vi "GetPower.vi"(6 "Calculation State in":T5, 8 "error in (no error)":errorcluster, 9 "Channel":T1, 10 "3-phase current waveform":waveform(dbl)[](array[waveform]), 11 "3-phase voltage waveform":waveform(dbl)[](array[waveform])) -> (0 "error out":errorcluster, 2 "power value":T6, 4 "Calculation State out":T5)   [LabVIEW 2017, in "McsaAnalysisFunctions.lvlib"]
uses:
  <vilib>/addons/InsightCM/Utilities/Analysis/MCSA/McsaAnalysisFunctions.lvlib
  <vilib>/addons/InsightCM/Utilities/Analysis/MCSA/controls/MotorCalculationCache.ctl
  <vilib>/addons/Electrical Power/Basic/Measurement/subVIs/basic_Power Value.ctl
  <vilib>/addons/InsightCM/Utilities/Analysis/MCSA/controls/TorqueLoadEfficiency.ctl
  <vilib>/addons/InsightCM/Utilities/Analysis/MCSA/controls/McsaChannel.ctl
  <vilib>/addons/InsightCM/Utilities/Analysis/Shared/controls/Feature.ctl
  <vilib>/addons/InsightCM/Utilities/Analysis/Shared/controls/AmplitudeScale.ctl
  <vilib>/addons/InsightCM/MessageBus/Base/controls/KeyValuePair.ctl
  <vilib>/addons/Electrical Power/Basic/NI_EP_Basic.lvlib
  <vilib>/addons/InsightCM/Utilities/Analysis/Shared/AnalysisHelper.lvlib
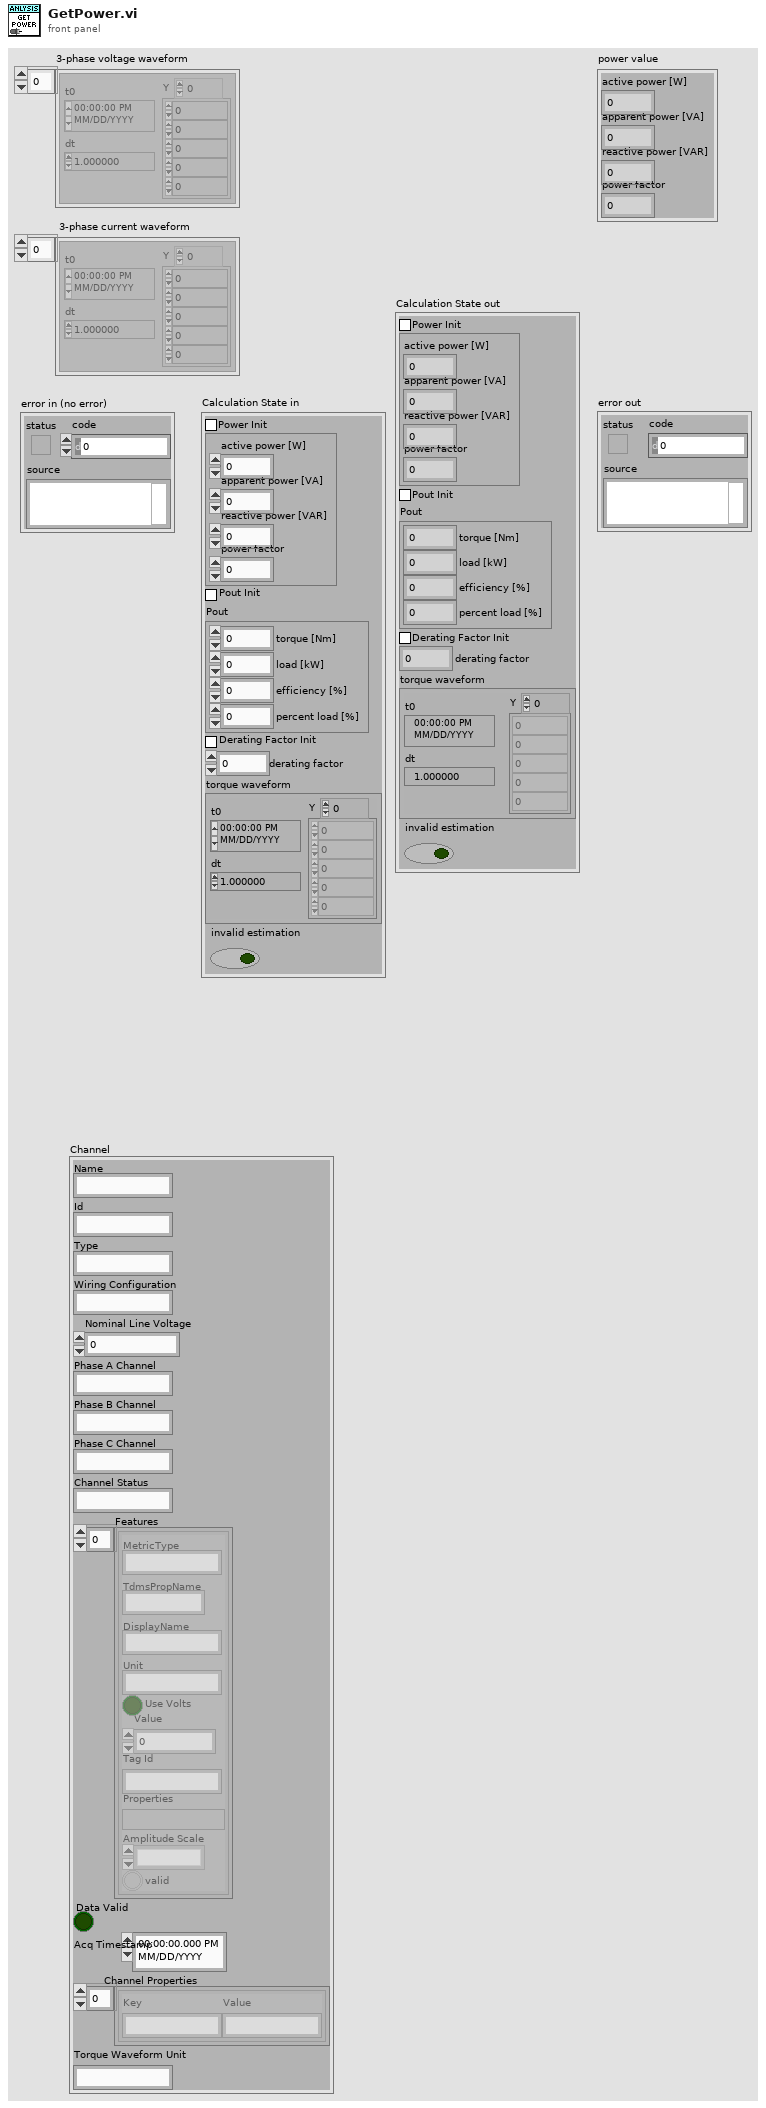
[diagram p1: front panel]
types:
  T1 = typedef "McsaAnalysisFunctions.lvlib/McsaChannel.ctl" = cluster{"Name":string, "Id":string, "Type":string, "Wiring Configuration":string, "Nominal Line Voltage":dbl, "Phase A Channel":string, "Phase B Channel":string, "Phase C Channel":string, "Channel Status":string, "Features":T2[], "Data Valid":bool, "Acq Timestamp":timestamp, "Channel Properties":T4[], "Torque Waveform Unit":string}
  T2 = typedef "AnalysisHelper.lvlib/Feature.ctl" = cluster{"MetricType":string, "TdmsPropName":string, "DisplayName":string, "Unit":string, "Use Volts":bool, "Value":dbl, "Tag Id":string, "Properties":variant, "Amplitude Scale":T3, "valid":bool}
  T3 = typedef "AnalysisHelper.lvlib/AmplitudeScale.ctl" = enum16{"rms", "peak", "pk-pk"}
  T4 = typedef "KeyValuePair.ctl" = cluster{"Key":string, "Value":string}
  T5 = typedef "McsaAnalysisFunctions.lvlib/MotorCalculationCache.ctl" = cluster{"Power Init":bool, "power value":T6, "Pout Init":bool, "Pout":T7, "Derating Factor Init":bool, "derating factor":sgl, "torque waveform":waveform(dbl), "invalid estimation":bool}
  T6 = typedef "NI_EP_Basic.lvlib/basic_Power Value.ctl" = cluster{"active power [W]":dbl, "apparent power [VA]":dbl, "reactive power [VAR]":dbl, "power factor":dbl}
  T7 = typedef "McsaAnalysisFunctions.lvlib/TorqueLoadEfficiency.ctl" = cluster{"torque [Nm]":dbl, "load [kW]":dbl, "efficiency [%]":dbl, "percent load [%]":dbl}
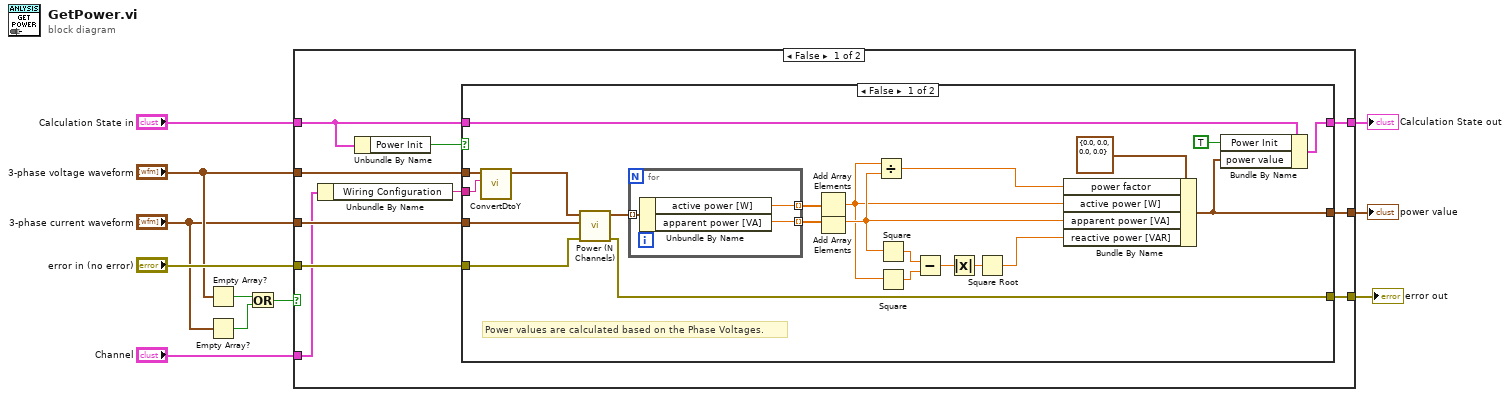
[diagram p0: block diagram]
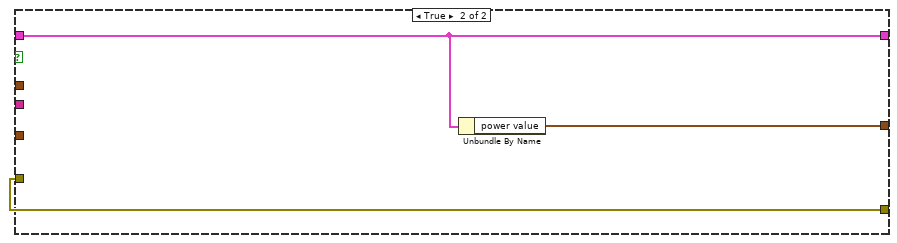
[diagram p2: hidden frame]
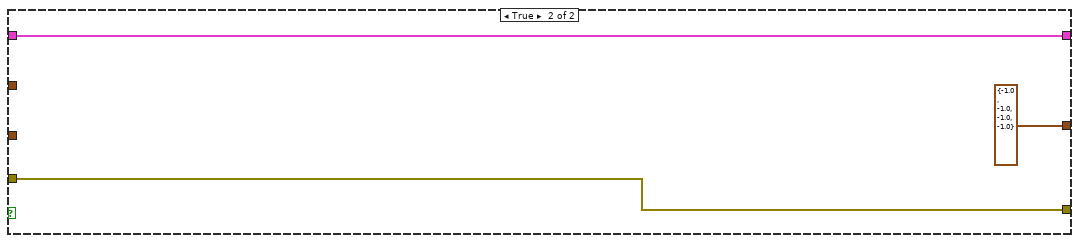
[diagram p3: hidden frame]
diagram:
  n1 = Empty Array?(array="3-phase voltage waveform") -> (empty?=w4:bool)
  n2 = Empty Array?(array="3-phase current waveform") -> (empty?=w3:bool)
  n3 = Or(x=w4, y=w3) -> (x .or. y?=w2:bool)
  n4 = case shown="False" w2 {
    tunnel: "Calculation State in" -> [w20 w52]
    tunnel: "3-phase voltage waveform" -> [w19 _]
    tunnel: "3-phase current waveform" -> [w18 _]
    tunnel: [w17 T6 {"active power [W]"=-1.0, "apparent power [VA]"=-1.0, "reactive power [VAR]"=-1.0, "power factor"=-1.0} ("power value")] -> w10
    tunnel: "error in (no error)" -> [w16 w50]
    tunnel: [w15 w50] -> w8
    tunnel: [w14 w52] -> w7
    tunnel: "Channel" -> [w13 _]
    frame False {
      n5 = Unbundle By Name(w13) -> ("Wiring Configuration"=w12:string)
      n6 = Unbundle By Name(w20) -> ("Power Init"=w21:bool)
      n7 = case shown="False" w21 {
        tunnel: w19 -> [w27 _]
        tunnel: [w29 w49] -> w17
        tunnel: w20 -> [w43 w48]
        tunnel: [w42 w48] -> w14
        tunnel: w18 -> [w23 _]
        tunnel: w16 -> [w26 w47]
        tunnel: [w25 w47] -> w15
        tunnel: w12 -> [w24 _]
        frame False {
          # "Power values are calculated based on the Phase Voltages."
          n8 = call <vilib>:"ConvertDtoY.vi"("Wiring Configuration"=w24, "voltage waveform"=w27) -> ("phase voltage waveform"=w22:waveform(dbl)[])  [unwired: 8 in, 1 out]
          n9 = call <vilib>:"Power (N Channels).vi"("error in (no error)"=w26, "current waveforms"=w23, "voltage waveforms"=w22) -> ("error out"=w25:errorcluster, "power values"=w40:T6[])  [unwired: 7 in]
          n10 = for {
            tunnel: w40 -> [w46] mode=indexing
            tunnel: [w45] -> w39 mode=indexing
            tunnel: [w44] -> w38 mode=indexing
            n11 = Unbundle By Name(w46) -> ("active power [W]"=w45:dbl, "apparent power [VA]"=w44:dbl)
          }
          n12 = Add Array Elements(numeric array=w39) -> (sum=w28:dbl)
          n13 = Add Array Elements(numeric array=w38) -> (sum=w31:dbl)
          n14 = Divide(x=w28, y=w31) -> (x/y=w32:dbl)
          n15 = Square(x=w31) -> (x^2=w35:dbl)
          n16 = Square(x=w28) -> (x^2=w34:dbl)
          n17 = Subtract(x=w35, y=w34) -> (x-y=w36:dbl)
          n18 = Absolute Value(x=w36) -> (abs(x)=w37:dbl)
          n19 = Square Root(x=w37) -> (sqrt(x)=w30:dbl)
          n20 = Bundle By Name(cluster=T6 {"active power [W]"=0.0, "apparent power [VA]"=0.0, "reactive power [VAR]"=0.0, "power factor"=0.0} ("power value"), "power factor"=w32, "active power [W]"=w28, "apparent power [VA]"=w31, "reactive power [VAR]"=w30) -> (w29:T6)
          n21 = Bundle By Name(cluster=w43, "Power Init"=TRUE ("Levels Init"), "power value"=w29) -> (w42:T5)
        }
        frame True {
          n22 = Unbundle By Name(w48) -> ("power value"=w49:T6)
        }
      }
    }
    frame True {
    }
  }
  "power value" <- w10
  "error out" <- w8
  "Calculation State out" <- w7
